vi "Handle Error.vi"(8 "error in (no error)":errorcluster, 11 "File Worker in":refnum<class "File Worker.lvclass">) -> (0 "error out":errorcluster, 2 "stop actor?":bool=TRUE, 3 "File Worker out":refnum<class "File Worker.lvclass">)   [LabVIEW 2025, in "File Worker.lvlib" / "File Worker.lvclass"]
doc: "<p>(<strong>Filename</strong>: <span class=\"dnl\">Actor Framework.lvlib:Actor.lvclass:Handle Error.vi</span>)</p>\n<p>Defines how the actor handles an error that occurred while processing a message. By default, this method does nothing except stop the actor.</p>"
uses:
  File Worker.lvclass
  File Worker.lvclass/File Worker.ctl
  <vilib>/MGI/Panel Manager/Panel Actor/Panel Actor/Panel Actor.lvclass
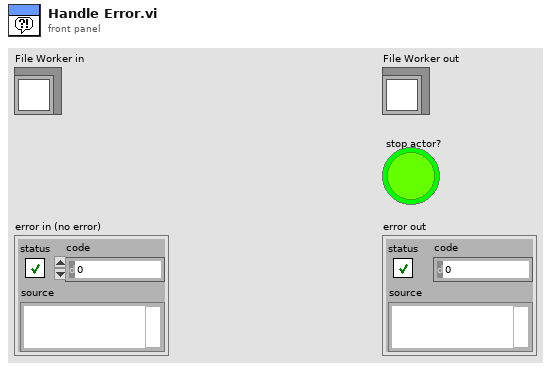
[diagram p1: front panel]
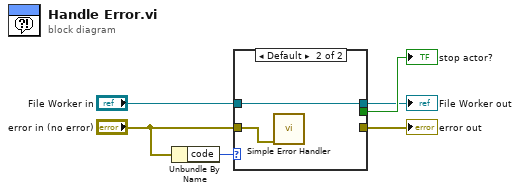
[diagram p0: block diagram]
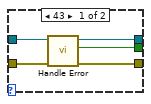
[diagram p2: hidden frame]
diagram:
  n1 = Unbundle By Name("error in (no error)") -> ("code"=w6:i32)
  n2 = case shown="Default" w6 {
    tunnel: [w11 _] -> w5
    tunnel: [w10 _] -> w4
    tunnel: [w9 w13] -> w3
    tunnel: "File Worker in" -> [w8 w13]
    tunnel: "error in (no error)" -> [w7 w12]
    frame 43 {
      n3 = call-parent "Handle Error.vi"("error in (no error)"=w7, "Actor in"=w8) -> ("error out"=w11:errorcluster, "stop actor?"=w10:bool, "Actor out"=w9:refnum<class "File Worker.lvclass">)  [unwired: 7 in]
    }
    frame Default {
      n4 = call <vilib>:"Simple Error Handler.vi"("error in (no error)"=w12) -> ()  [unwired: 4 in, 5 out]
    }
  }
  "File Worker out" <- w3
  "error out" <- w5
  "stop actor?" <- w4
